vi "FlatToRichnixnet_grpc_EnetFrameRequest.vi"(5 "OutputClusterType":T1, 11 "InputCluster":T3) -> (3 "OutputCluster":T1)   [LabVIEW 2025, in "xnet-grpc_client.lvlib"]
uses:
  nixnet_grpc_EnetFrameRequest_Flat.ctl
  nixnet_grpc_EnetFrameType.ctl
  nixnet_grpc_EnetFlags.ctl
  nixnet_grpc_EnetFrameRequest.ctl
  nixnet_grpc_EnetFrameRequest_type_enum/nixnet_grpc_EnetFrameRequest_type_enum.lvclass
  xnet-grpc_client.lvlib
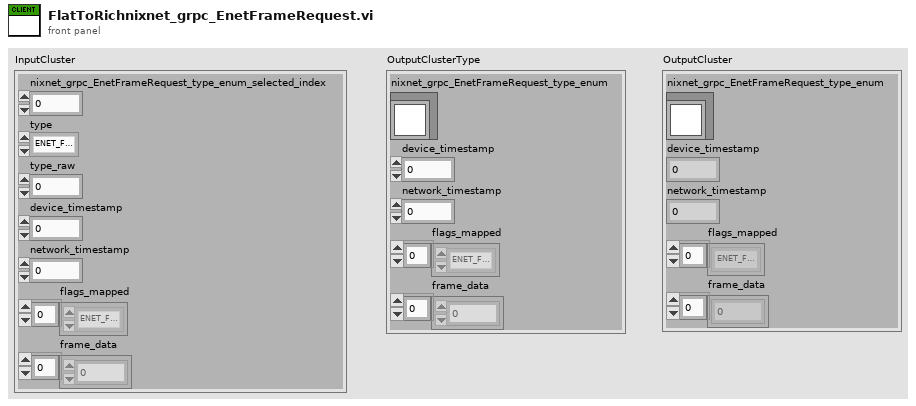
[diagram p1: front panel]
types:
  T1 = typedef "xnet-grpc_client.lvlib/nixnet_grpc_EnetFrameRequest.ctl" = cluster{"nixnet_grpc_EnetFrameRequest_type_enum":refnum<class "nixnet_grpc_EnetFrameRequest_type_enum.lvclass">, "device_timestamp":u64, "network_timestamp":u64, "flags_mapped":T2[], "frame_data":u8[]}
  T2 = typedef "xnet-grpc_client.lvlib/nixnet_grpc_EnetFlags.ctl" = enum32{"ENET_FLAGS_UNSPECIFIED", "ENET_FLAGS_TRANSMIT", "ENET_FLAGS_RECEIVE", "ENET_FLAGS_NETWORK_SYNCED", "ENET_FLAGS_ERROR"}
  T3 = typedef "xnet-grpc_client.lvlib/nixnet_grpc_EnetFrameRequest_Flat.ctl" = cluster{"nixnet_grpc_EnetFrameRequest_type_enum_selected_index":i32, "type":T4, "type_raw":u32, "device_timestamp":u64, "network_timestamp":u64, "flags_mapped":T2[], "frame_data":u8[]}
  T4 = typedef "xnet-grpc_client.lvlib/nixnet_grpc_EnetFrameType.ctl" = enum32{"ENET_FRAME_TYPE_DATA", "ENET_FRAME_TYPE_DELAY", "ENET_FRAME_TYPE_FUTURE_TIME_WAIT"}
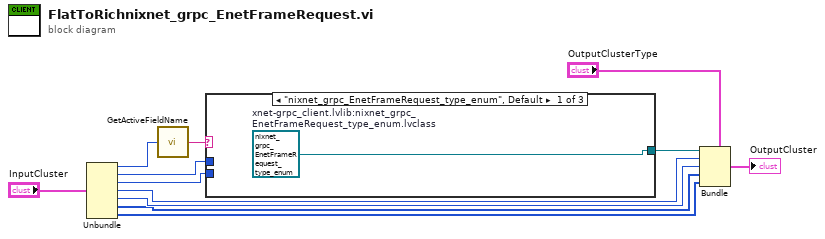
[diagram p0: block diagram]
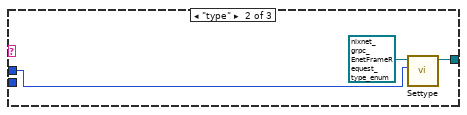
[diagram p2: hidden frame]
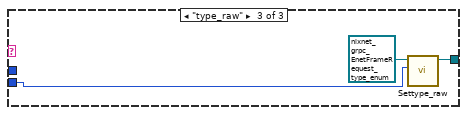
[diagram p3: hidden frame]
diagram:
  n1 = Unbundle "Unbundle"("InputCluster") -> ("nixnet_grpc_EnetFrameRequest_type_enum_selected_index"=w9:i32, "type"=w6:T4, "type_raw"=w5:u32, "device_timestamp"=w4:u64, "network_timestamp"=w3:u64, "flags_mapped"=w2:T2[], "frame_data"=w1:u8[])
  n2 = call "GetActiveFieldName.vi"("protobuf index"=w9) -> ("oneof field name"=w8:string)
  n3 = case "nixnet_grpc_EnetFrameRequest_type_enum" shown="\"nixnet_grpc_EnetFrameRequest_type_enum\", Default" w8 {
    tunnel: [w13 w15 w18] -> w7
    tunnel: w6 -> [_ w16 _]
    tunnel: w5 -> [_ _ w19]
    frame "nixnet_grpc_EnetFrameRequest_type_enum", Default {
      w13 = refnum<class "nixnet_grpc_EnetFrameRequest_type_enum.lvclass"> refnum  # xnet-grpc_client.lvlib:nixnet_grpc_EnetFrameRequest_type_enum.lvclass
    }
    frame "type" {
      n4 = call "Settype.vi"("Set_Val"=w16, "OneOfTemplate in"=refnum<class "nixnet_grpc_EnetFrameRequest_type_enum.lvclass"> refnum) -> ("OneOfTemplate out"=w15:refnum<class "nixnet_grpc_EnetFrameRequest_type_enum.lvclass">)  [unwired: 8 in, 1 out]
    }
    frame "type_raw" {
      n5 = call "Settype_raw.vi"("Set_Val"=w19, "OneOfTemplate in"=refnum<class "nixnet_grpc_EnetFrameRequest_type_enum.lvclass"> refnum) -> ("OneOfTemplate out"=w18:refnum<class "nixnet_grpc_EnetFrameRequest_type_enum.lvclass">)  [unwired: 8 in, 1 out]
    }
  }
  n6 = Bundle "Bundle"(cluster="OutputClusterType", "nixnet_grpc_EnetFrameRequest_type_enum"=w7, "device_timestamp"=w4, "network_timestamp"=w3, "flags_mapped"=w2, "frame_data"=w1) -> (→"OutputCluster":T1)
